vi "Get Menu Item Info.vi"(8 "error in (no error)":errorcluster, 10 "item tag":string, 11 "Menu in":refnum<class "Menu.lvclass">) -> (0 "error out":errorcluster, 1 "enabled":bool, 2 "item name":string, 3 "Menu out":refnum<class "Menu.lvclass">, 4 "checked":bool, 5 "submenu tags":string[](array[string]), 6 "short cut":T1, 7 "Picture":refnum<class "Image.lvclass">)   [LabVIEW 2021, in "Menu.lvlib" / "Menu.lvclass"]
uses:
  Menu.lvclass
  Menu.lvclass/Menu.ctl
  <vilib>/Utility/miscctls.llb/LVMenuShortCut.ctl
  Picture2D/src/Picture/Image.lvclass
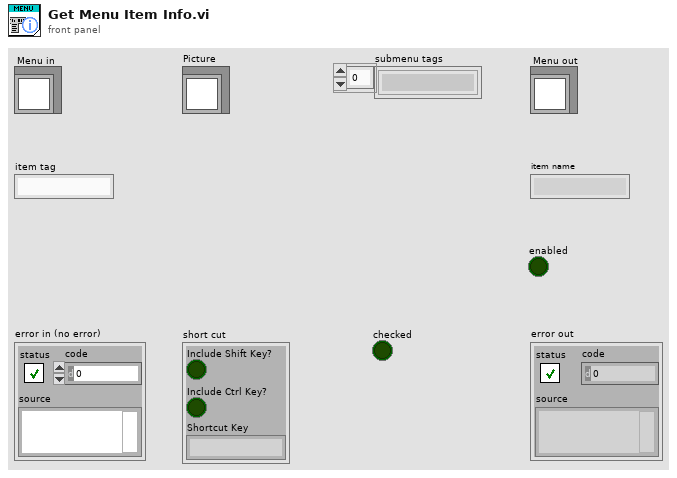
[diagram p1: front panel]
types:
  T1 = typedef "LVMenuShortCut.ctl" = cluster{"Include Shift Key?":bool, "Include Ctrl Key?":bool, "Shortcut Key":string}
  T2 = typedef "Menu.lvlib/Menu.lvclass/Data.ctl" = cluster{"MenuMap":map{string, T3}, "PictRef":refnum<vi>, "MenuSelectionEvent":refnum<user-event>, "TopMenuSpacing":i32, "MenuSpacing":i32, "CloseEvent":refnum<user-event>, "TR_ManageMenuRef":refnum<vi>, "MenuColors":T4, "RTMPath":path, "RTMVIReference":refnum<vi>, "RTMMenuReference":refnum<k9>, "CtlRef":refnum<vi>, "User-Specified Font":refnum<class "Font.lvclass">, "Desired Font":enum16{"User-specified Font", "Application Font", "System Font", "Dialog Font"}, "SubMenuIcon":T5, "SubMenuIconClosed":refnum<class "Picture2D.lvclass">, "SubMenuIconOpened":refnum<class "Picture2D.lvclass">}
  T3 = typedef "Menu.lvlib/Menu.lvclass/MenuItems.ctl" = cluster{"Item Name":string, "Short Cut":T1, "Checked":bool, "Enable":bool, "After item":string, "Item Tags":string[], "Item Names":string[], "Picture":refnum<class "Image.lvclass">, "Hilite Picture":refnum<class "Image.lvclass">, "Displayed":bool}
  T4 = typedef "Menu.lvlib/Menu.lvclass/MenuColors.ctl" = cluster{"Text":refnum<class "Color.lvclass">, "HiliteText":refnum<class "Color.lvclass">, "Background":refnum<class "Color.lvclass">, "BorderColor":refnum<class "Color.lvclass">, "Hilite":refnum<class "Color.lvclass">}
  T5 = typedef "Menu.lvlib/Menu.lvclass/SubMenuIcon.ctl" = enum16{"LabVIEW", "Windows", "Custom"}
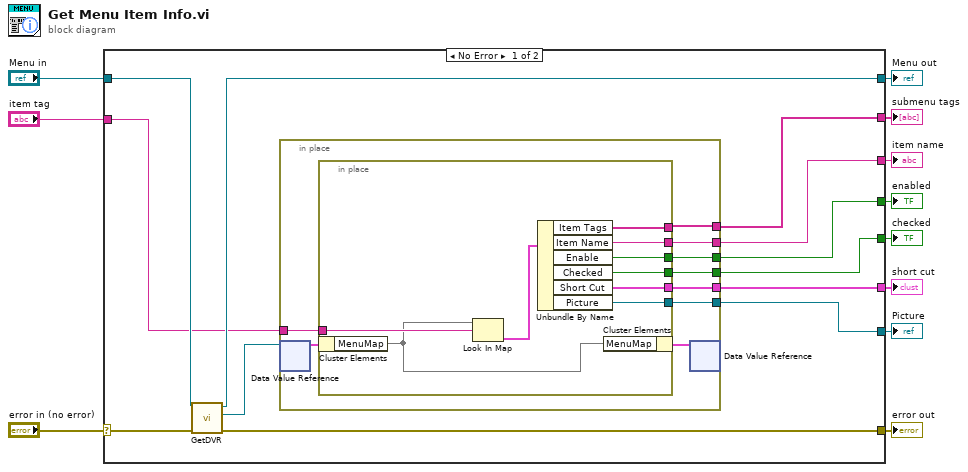
[diagram p0: block diagram]
diagram:
  n1 = case shown="No Error" "error in (no error)" {
    selector: "error in (no error)" -> [w23 w43]
    tunnel: [w22 w43] -> w10
    tunnel: [w21 w42] -> w8
    tunnel: "Menu in" -> [w20 w42]
    tunnel: "item tag" -> [w18 _]
    tunnel: [w16 _] -> w6
    tunnel: [w17 _] -> w5
    tunnel: [w13 _] -> w4
    tunnel: [w14 _] -> w3
    tunnel: [w15 _] -> w2
    tunnel: [w12 _] -> w1
    frame No Error {
      n2 = call "GetDVR.vi"("error in (no error)"=w23, "Menu in"=w20) -> ("error out"=w22:errorcluster, "DVR"=w19:refnum<data-value>, "Menu out"=w21:refnum<class "Menu.lvclass">)  [unwired: 7 in]
      n3 = in-place {
        in-place-border: w18 -> [w30]
        in-place-border: [w29] -> w17
        in-place-border: [w28] -> w16
        in-place-border: [w27] -> w15
        in-place-border: [w26] -> w14
        in-place-border: [w25] -> w13
        in-place-border: [w24] -> w12
        n4 = in-place-dvr #1(w19) -> (w32:T2)  [unwired: 1 out]
        n5 = in-place {
          in-place-border: w30 -> [w41]
          in-place-border: [w39] -> w29
          in-place-border: [w38] -> w28
          in-place-border: [w37] -> w27
          in-place-border: [w36] -> w26
          in-place-border: [w35] -> w25
          in-place-border: [w33] -> w24
          n6 = in-place-cluster #2(w32) -> ("MenuMap"=w34:map{string, T3})
          n7 = Look In Map(map=w34, key=w41) -> (value=w40:T3)  [unwired: 1 in, 1 out]
          n8 = Unbundle By Name(w40) -> ("Item Tags"=w38:string[], "Item Name"=w39:string, "Enable"=w37:bool, "Checked"=w36:bool, "Short Cut"=w35:T1, "Picture"=w33:refnum<class "Image.lvclass">)
          n9 = in-place-cluster #2("MenuMap"=w34) -> (w31:T2)
        }
        n10 = in-place-dvr #1(w31) -> ()  [unwired: 2 out]
      }
    }
    frame Error {
    }
  }
  "error out" <- w10
  "Menu out" <- w8
  "submenu tags" <- w6
  "item name" <- w5
  "short cut" <- w4
  "checked" <- w3
  "enabled" <- w2
  "Picture" <- w1
